vi "Populate Array Channel.vi"(8 "error in (no error)":errorcluster, 10 "Channel Refnum":T2 format="%.0x", 11 "Elements":T1[](array[typedef])) -> (0 "error out":errorcluster)   [LabVIEW 2018, in "Instrument Addon Scripting API.lvlib"]
uses:
  Instrument Addon Scripting API.lvlib
  <vilib>/NI Veristand/Custom Device API/Custom Device Item Ref.ctl
  TypeDefs/Array Element.ctl
  <vilib>/NI Veristand/Custom Device API/Custom Device Channel.ctl
  <vilib>/NI Veristand/Custom Device API/Custom Device Channel Type.ctl
  Addon/Addon Shared/SubVIs/Constants.vi
  <vilib>/NI Veristand/Custom Device API/Custom Device API.lvlib
  Addon/Addon Shared/Instrument Addon Shared.lvlib
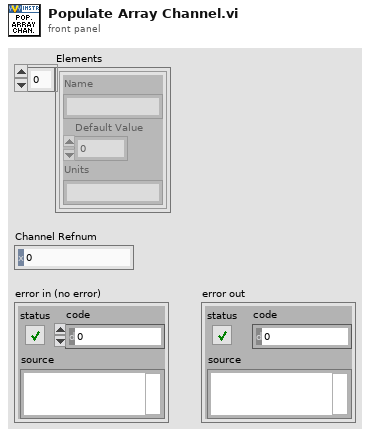
[diagram p1: front panel]
types:
  T1 = typedef "Instrument Addon Scripting API.lvlib/Array Element.ctl" = cluster{"Name":string, "Default Value":dbl, "Units":string}
  T2 = typedef "Custom Device API.lvlib/Custom Device Item Ref.ctl" = u64
  T3 = typedef "Custom Device API.lvlib/Custom Device Channel.ctl" = cluster{"Type":T4, "Units":string, "Default Value":dbl, "Faultable":bool, "Scalable":bool}
  T4 = typedef "Custom Device API.lvlib/Custom Device Channel Type.ctl" = enum16{"Input", "Output"}
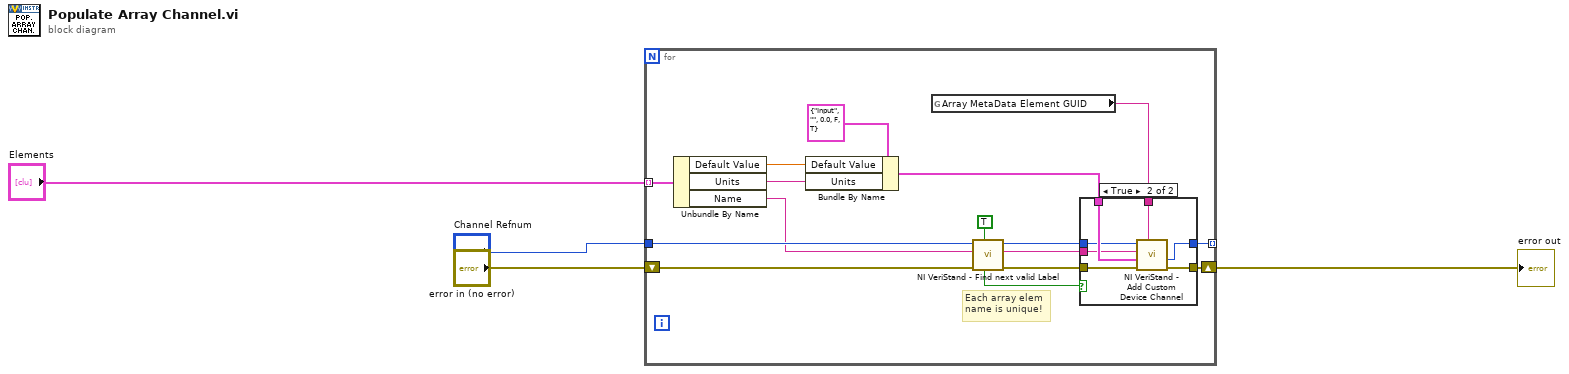
[diagram p0: block diagram]
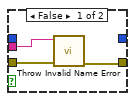
[diagram p2: hidden frame]
diagram:
  n1 = for {
    shift-right: [w20] -> w4
    shift-left: "error in (no error)" -> [w10]
    tunnel: "Elements" -> [w15] mode=indexing
    tunnel: "Channel Refnum" -> [w11]
    tunnel: [w17] -> _ mode=indexing
    # "Each array elem\nname is unique!"
    n2 = Unbundle By Name(w15) -> ("Default Value"=w14:dbl, "Units"=w13:string, "Name"=w9:string)
    n3 = Bundle By Name(cluster=T3 {"Type"=enum."Input", "Units"="", "Default Value"=0.0, "Faultable"=FALSE, "Scalable"=TRUE} ("Channel"), "Default Value"=w14, "Units"=w13) -> (w18:T3)
    n4 = global read "Constants.vi" "Array MetaData Element GUID"() -> (w16:string)
    n5 = call <vilib>:"NI VeriStand - Find next valid Label.vi"("Try requested Label only?"=TRUE, "error in (no error)"=w10, "Label"=w9, "Item Ref in"=w11) -> ("error out"=w6:errorcluster, "Label out"=w7:string, "Item Ref out"=w8:T2, "Requested label not in use?"=w5:bool)  [unwired: 3 in, 1 out]
    n6 = case shown="True" w5 {
      tunnel: [w21 w30] -> w20
      tunnel: w18 -> [_ w29]
      tunnel: [_ w24] -> w17
      tunnel: w16 -> [_ w28]
      tunnel: w8 -> [_ w27]
      tunnel: w7 -> [w22 w26]
      tunnel: w6 -> [w23 w25]
      frame False {
        n7 = call "Throw Invalid Name Error.vi"("error in (no error)"=w23, "Name"=w22) -> ("error out"=w21:errorcluster)  [unwired: 9 in]
      }
      frame True {
        n8 = call <vilib>:"NI VeriStand - Add Custom Device Channel.vi"("GUID (Default Channel)"=w28, "error in (no error)"=w25, "Channel"=w29, "Channel Name"=w26, "Parent Ref in"=w27) -> ("error out"=w30:errorcluster, "Channel Ref"=w24:T2)  [unwired: 3 in, 2 out]
      }
    }
  }
  "error out" <- w4
